vi "TestTon.vi"() -> ()   [LabVIEW 2022 SP3, in "BinarySignalProcessClass.lvclass"]
uses:
  BinarySignalProcessClass.lvclass
panel:
  out "elapsed time (ms)":i32
  out "Waveform Chart 2":i32(graph)
  in  "stop":bool
  out "Waveform Chart":i32(graph)
  in  "input":bool
  in  "Ton":i32=1000
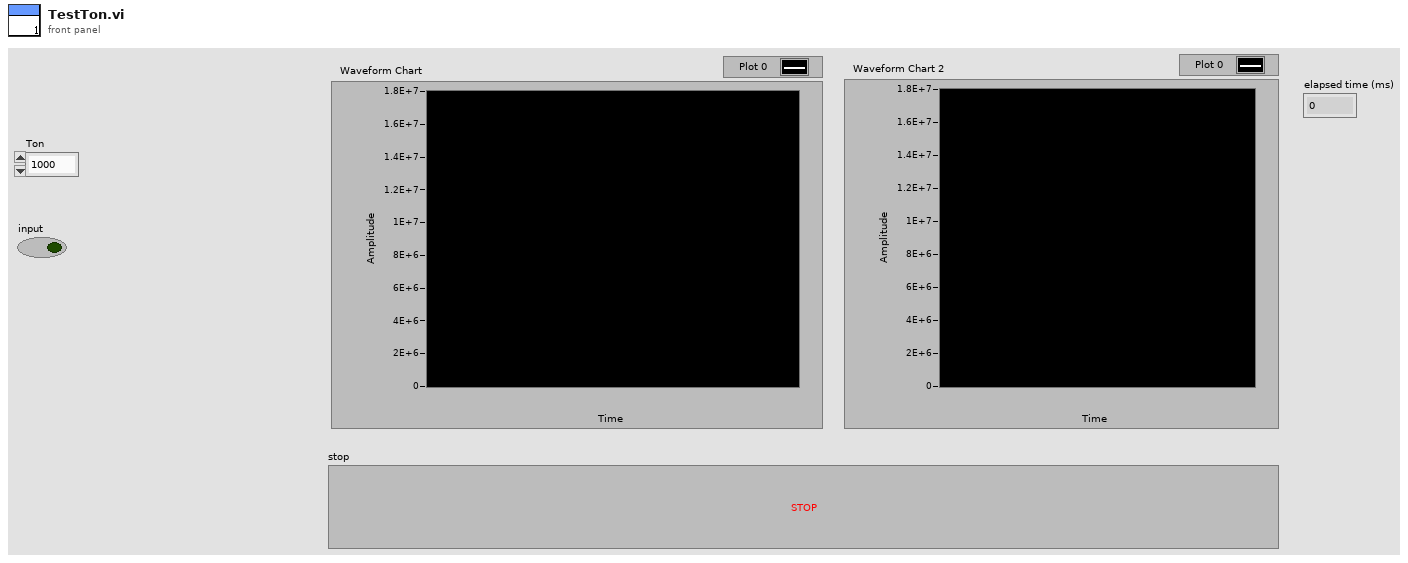
[diagram p1: front panel]
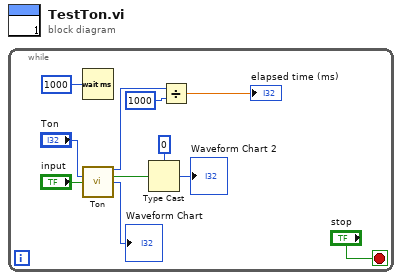
[diagram p0: block diagram]
diagram:
  n1 = while {
    stop <- "stop" stop-if-true
    n2 = Wait (ms)(milliseconds to wait=u32 1000) -> ()  [unwired: 1 out]
    n3 = call "Ton.vi"("Ton"="Ton", "input"="input") -> ("elapsed time (ms)"=w3:i32, "Pulse"=w5:bool, "on"=→"Waveform Chart":i32)  [unwired: 10 in, 1 out]
    n4 = Type Cast(type=0, x=w5) -> (*(type *) &x=→"Waveform Chart 2":i32)
    n5 = Divide(x=w3, y=1000) -> (x/y=→"elapsed time (ms)":dbl)
  }
